vi "Divide Polynomials (DBL).vi"(8 "threshold type":T1 items=["Absolute Value", "Relative Value"], 9 "threshold":dbl, 10 "Q(x)":dbl[](array[numeric]), 11 "P(x)":dbl[](array[numeric])) -> (0 "error":i32, 2 "Remainder":dbl[](array[numeric]), 3 "P(x)/Q(x)":dbl[](array[numeric]))   [LabVIEW 2010, in "NI_AALPro.lvlib"]
doc: "Divides polynomial <B>P(x)</B> by polynomial <B>Q(x)</B>. The data types you wire to the <B>P(x)</B> and <B>Q(x)</B> inputs determine the polymorphic instance to use."
uses:
  NI_AALPro.lvlib
  Remove Zero Threshold Type.ctl
  Remove Zero Coefficients (DBL).vi
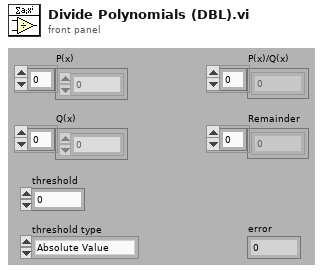
[diagram p1: front panel]
types:
  T1 = typedef "NI_AALPro.lvlib/Remove Zero Threshold Type.ctl" = u16
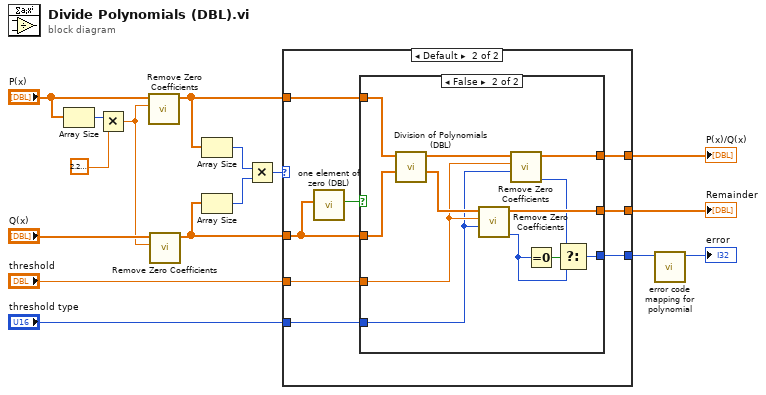
[diagram p0: block diagram]
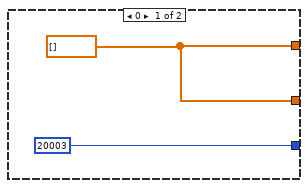
[diagram p2: hidden frame]
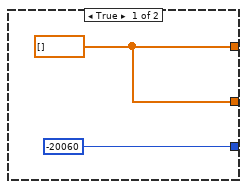
[diagram p3: hidden frame]
diagram:
  n1 = Array Size(array="P(x)") -> (size(s)=w16:i32)
  n2 = Multiply(x=w16, y=2.220446049250313e-16) -> (x*y=w9:dbl)
  n3 = call-poly "Remove Zero Coefficients.vi"("threshold"=w9, "P(x) In"="P(x)") -> ("P(x) Out"=w12:dbl[])  [unwired: 7 in, 2 out]
  n4 = call-poly "Remove Zero Coefficients.vi"("threshold"=w9, "P(x) In"="Q(x)") -> ("P(x) Out"=w8:dbl[])  [unwired: 7 in, 2 out]
  n5 = Array Size(array=w12) -> (size(s)=w14:i32)
  n6 = Array Size(array=w8) -> (size(s)=w13:i32)
  n7 = Multiply(x=w14, y=w13) -> (x*y=w11:i32)
  n8 = case shown="Default" w11 {
    tunnel: w12 -> [_ w26]
    tunnel: w8 -> [_ w22]
    tunnel: [w18 w25] -> w7
    tunnel: [w18 w24] -> w6
    tunnel: [20003 ("empty array") w23] -> w5
    tunnel: "threshold" -> [_ w20]
    tunnel: "threshold type" -> [_ w19]
    frame 0 {
      w18 = dbl[] []
    }
    frame Default {
      n9 = call "one element of zero (DBL).vi"("Array in"=w22) -> ("equal [0]?"=w21:bool)  [unwired: 10 in]
      n10 = case shown="False" w21 {
        tunnel: w26 -> [_ w40]
        tunnel: w22 -> [_ w39]
        tunnel: [w28 w37] -> w25
        tunnel: [w28 w35] -> w24
        tunnel: [-20060 ("divide by zero") w31] -> w23
        tunnel: w20 -> [_ w30]
        tunnel: w19 -> [_ w29]
        frame True {
          w28 = dbl[] []
        }
        frame False {
          n11 = call "Division of Polynomials (DBL).vi"("q"=w39, "p"=w40) -> ("rest"=w36:dbl[], "p/q"=w38:dbl[])  [unwired: 8 in]
          n12 = call-poly "Remove Zero Coefficients.vi"("threshold type"=w29, "threshold"=w30, "P(x) In"=w36) -> ("error"=w32:i32, "P(x) Out"=w35:dbl[])  [unwired: 6 in, 1 out]
          n13 = call-poly "Remove Zero Coefficients.vi"("threshold type"=w29, "threshold"=w30, "P(x) In"=w38) -> ("error"=w33:i32, "P(x) Out"=w37:dbl[])  [unwired: 6 in, 1 out]
          n14 = Equal To 0?(x=w32) -> (x = 0?=w34:bool)
          n15 = Select(t=w33, s=w34, f=w32) -> (s? t:f=w31:i32)
        }
      }
    }
  }
  "Remainder" <- w6
  "P(x)/Q(x)" <- w7
  n16 = call "error code mapping for polynomial.vi"("error in"=w5) -> ("error out"=→"error":i32)  [unwired: 10 in]
